vi "DOS cmd.vi"(8 "错误输入（无错误）":errorcluster) -> (0 "error out":errorcluster caption="错误输出")   [LabVIEW 2016, in "update.lvlib"]
uses:
  update.lvlib
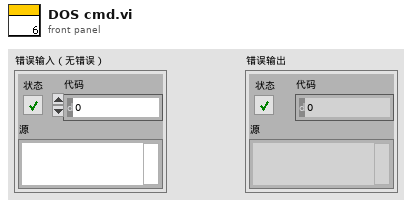
[diagram p1: front panel]
types:
  T1 = enum16{"open", "replace", "create", "open or create", "replace or create", "replace or create with confirmation"}
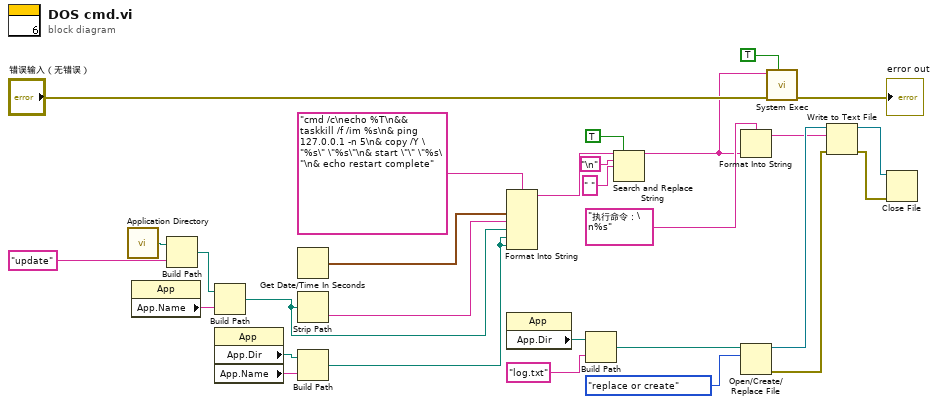
[diagram p0: block diagram]
diagram:
  n1 = call <vilib>:"Application Directory.vi"() -> ("Application Directory"=w14:path)
  n2 = property class="App"() -> ("App.Name"=w11:string)  [unwired: 2 in, 2 out]
  n3 = Build Path(base path=w14, name or relative path="update" ("名称或相对路径")) -> (appended path=w12:path)
  n4 = Build Path(base path=w12, name or relative path=w11) -> (appended path=w8:path)
  n5 = property class="App"() -> ("App.Dir"=w10:path, "App.Name"=w9:string)  [unwired: 2 in, 2 out]
  n6 = Get Date/Time In Seconds() -> (seconds since 1Jan1904=w15:timestamp)
  n7 = Strip Path(path=w8) -> (name=w16:string)  [unwired: 1 out]
  n8 = Build Path(base path=w10, name or relative path=w9) -> (appended path=w7:path)
  n9 = Format Into String(format string="cmd /c\necho %T\n&& taskkill /f /im %s\n& ping 127.0.0.1 -n 5\n& copy /Y \"%s\" \"%s\"\n& start \"\" \"%s\"\n& echo restart complete" ("文本"), w15, w16, w8, w7, w7) -> (resulting string=w4:string)  [unwired: 2 in, 1 out]
  n10 = property class="App"() -> ("App.Dir"=w23:path)  [unwired: 2 in, 2 out]
  n11 = Build Path(base path=w23, name or relative path="log.txt" ("名称或相对路径")) -> (appended path=w21:path)
  n12 = Search and Replace String(replace all?=TRUE ("替换全部？(F)"), input string=w4, search string="\n", replace string=" " ("替换字符串(\"\")")) -> (result string=w1:string)  [unwired: 4 in, 3 out]
  n13 = Format Into String(format string="执行命令：\n%s" ("格式字符串"), w1) -> (resulting string=w18:string)  [unwired: 2 in, 1 out]
  n14 = Open/Create/Replace File(file path (use dialog)=w21, operation (0:open)=T1."replace or create" ("操作(0:open)")) -> (refnum out=w24:refnum<file>, error out=w27:errorcluster)  [unwired: 4 in, 1 out]
  n15 = call <vilib>:"System Exec.vi"("wait until completion? (T)"=TRUE, "error in (no error)"="错误输入（无错误）", "command line"=w1) -> ("error out"=→"error out":errorcluster)  [unwired: 5 in, 3 out]
  n16 = Write to Text File(file (use dialog)=w24, text=w18, error in=w27) -> (refnum out=w25:refnum<file>, error out=w26:errorcluster)  [unwired: 1 in, 1 out]
  n17 = Close File(refnum=w25, error in=w26) -> ()  [unwired: 2 out]
